vi "Read Config.vi"(8 "error in (no error)":errorcluster caption="entrée d'erreur (pas d'erreur)", 11 "GeneralFunctionality en entrée":refnum<class "GeneralFunctionality.lvclass">) -> (0 "error out":errorcluster caption="sortie d'erreur", 2 "Config.lvclass":refnum<class "Config.lvclass">, 3 "GeneralFunctionality en sortie":refnum<class "GeneralFunctionality.lvclass">)   [LabVIEW 2020, in "GeneralFunctionality.lvclass"]
uses:
  GeneralFunctionality.lvclass
  Config/Config.lvclass
  GeneralFunctionality.lvclass/GeneralFunctionality.ctl
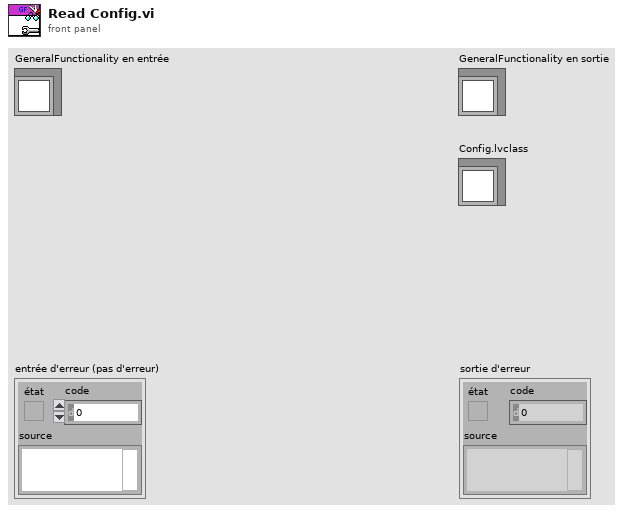
[diagram p1: front panel]
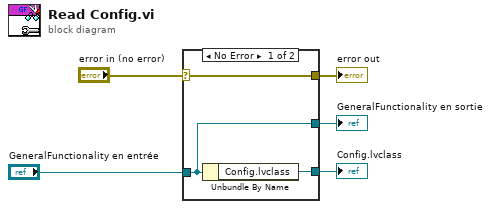
[diagram p0: block diagram]
diagram:
  n1 = case shown="No Error" "error in (no error)" {
    selector: "error in (no error)" -> [w8 w9]
    tunnel: [w8 w9] -> w4
    tunnel: [w7 w10] -> w2
    tunnel: "GeneralFunctionality en entrée" -> [w7 w10]
    tunnel: [w6 _] -> w1
    frame No Error {
      n2 = Unbundle By Name(w7) -> ("Config.lvclass"=w6:refnum<class "Config.lvclass">)
    }
    frame Error {
    }
  }
  "error out" <- w4
  "GeneralFunctionality en sortie" <- w2
  "Config.lvclass" <- w1
